vi "Clear DTC FIFOs.vi"(11 "Simulated Addresses":T1[](array[typedef]) {"Simulated Addresses"."J1939 XNET Settings"."Name" format="%.0x"; "Simulated Addresses"."DM1 Data"."Data Reference" format="%.0x"; "Simulated Addresses"."DM1 Enable?"."Data Reference" format="%.0x"; "Simulated Addresses"."DM2 Data"."Data Reference" format="%.0x"; "Simulated Addresses"."DM2 Enable?"."Data Reference" format="%.0x"}) -> ()   [LabVIEW 2015, in "J1939 Addon Engine.lvlib"]
uses:
  J1939 Addon Engine.lvlib
  Types/Simulated Settings.ctl
  Shared/Types/Compiled Simulated Settings.ctl
  Shared/Types/Monitor Settings.ctl
  <vilib>/NI Veristand/Custom Device API/Block Data Reference.ctl
  <vilib>/NI Veristand/Custom Device API/Data Reference.ctl
  Types/DTC FIFOs.ctl
  <vilib>/NI VeriStand/Custom Device API/Custom Device API.lvlib
  Shared/J1939 Addon Shared.lvlib
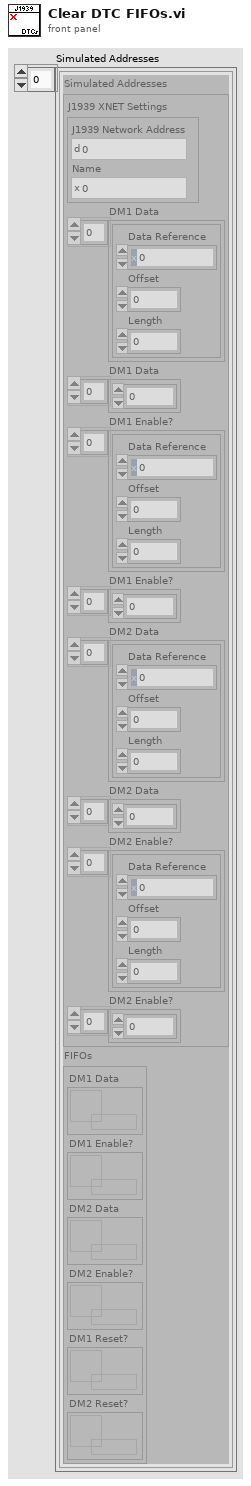
[diagram p1: front panel]
types:
  T1 = typedef "J1939 Addon Engine.lvlib/Simulated Settings.ctl" = cluster{"Simulated Addresses":T2, "FIFOs":T6}
  T2 = typedef "J1939 Addon Shared.lvlib/Compiled Simulated Settings.ctl" = cluster{"J1939 XNET Settings":T3, "DM1 Data":T4[], "DM1 Data":dbl[], "DM1 Enable?":T4[], "DM1 Enable?":dbl[], "DM2 Data":T4[], "DM2 Data":dbl[], "DM2 Enable?":T4[], "DM2 Enable?":dbl[]}
  T3 = typedef "J1939 Addon Shared.lvlib/Monitor Settings.ctl" = cluster{"J1939 Network Address":u8, "Name":u64}
  T4 = typedef "Custom Device API.lvlib/Block Data Reference.ctl" = cluster{"Data Reference":T5, "Offset":u64, "Length":u64}
  T5 = typedef "Custom Device API.lvlib/Data Reference.ctl" = i32
  T6 = typedef "J1939 Addon Engine.lvlib/DTC FIFOs.ctl" = cluster{"DM1 Data":refnum<k33>, "DM1 Enable?":refnum<k33>, "DM2 Data":refnum<k33>, "DM2 Enable?":refnum<k33>, "DM1 Reset?":refnum<k33>, "DM2 Reset?":refnum<k33>}
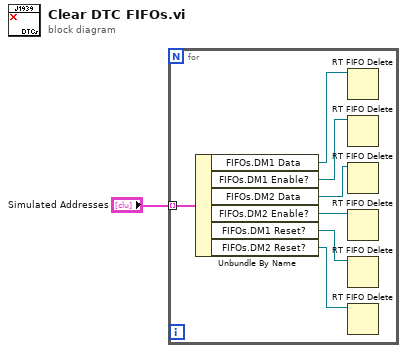
[diagram p0: block diagram]
diagram:
  n1 = for {
    tunnel: "Simulated Addresses" -> [w8] mode=indexing
    n2 = Unbundle By Name(w8) -> ("FIFOs.DM1 Data"=w7:refnum<k33>, "FIFOs.DM1 Enable?"=w6:refnum<k33>, "FIFOs.DM2 Data"=w5:refnum<k33>, "FIFOs.DM2 Enable?"=w4:refnum<k33>, "FIFOs.DM1 Reset?"=w3:refnum<k33>, "FIFOs.DM2 Reset?"=w2:refnum<k33>)
    n3 = RT FIFO Delete(0:w7) -> ()  [unwired: 2 in, 1 out]
    n4 = RT FIFO Delete(0:w6) -> ()  [unwired: 2 in, 1 out]
    n5 = RT FIFO Delete(0:w5) -> ()  [unwired: 2 in, 1 out]
    n6 = RT FIFO Delete(0:w4) -> ()  [unwired: 2 in, 1 out]
    n7 = RT FIFO Delete(0:w3) -> ()  [unwired: 2 in, 1 out]
    n8 = RT FIFO Delete(0:w2) -> ()  [unwired: 2 in, 1 out]
  }
